vi "Error_Detection.vi"(7 "Current State":string, 8 "error in (no error)":errorcluster, 11 "Msg In":string[](array[string])) -> (0 "error out":errorcluster, 3 "Msg Out":string[](array[string]))   [LabVIEW 2010]
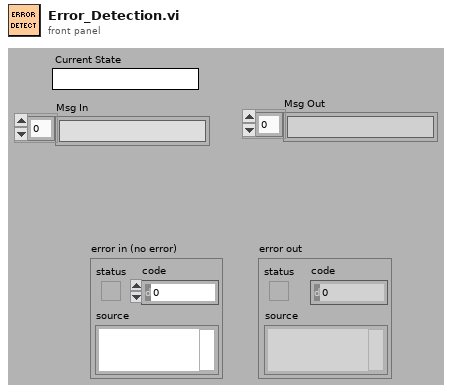
[diagram p1: front panel]
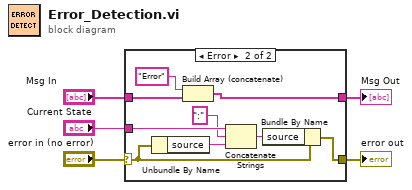
[diagram p0: block diagram]
diagram:
  n1 = case shown="Error" "error in (no error)" {
    selector: "error in (no error)" -> [w6 w10]
    tunnel: "Current State" -> [_ w13]
    tunnel: "Msg In" -> [w7 w16]
    tunnel: [w7 w15] -> w2
    tunnel: [w6 w8] -> w1
    frame No Error {
    }
    frame Error {
      n2 = Unbundle By Name(w10) -> ("source"=w11:string)
      n3 = Build Array (concatenate)("Error", w16) -> (w15:string[])
      n4 = Concatenate Strings(w13, ":" ("string"), w11) -> (w9:string)
      n5 = Bundle By Name(cluster=w10, "source"=w9) -> (w8:errorcluster)
    }
  }
  "error out" <- w1
  "Msg Out" <- w2
